vi "read position.vi"(8 "error in (no error)":errorcluster, 11 "CL57RS in":refnum<class "CL57RS.lvclass">) -> (0 "error out":errorcluster, 2 "Angle":dbl, 3 "CL57RS out":refnum<class "CL57RS.lvclass">)   [LabVIEW 2025, in "Motor.lvlib" / "CL57RS.lvclass"]
uses:
  CL57RS.lvclass
  CL57RS.lvclass/CL57RS.ctl
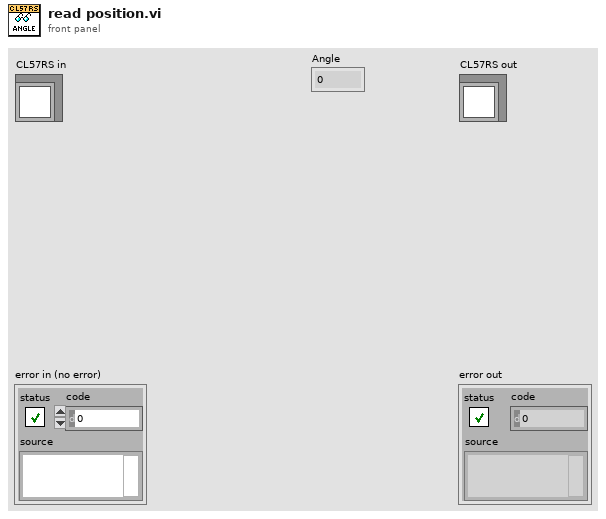
[diagram p1: front panel]
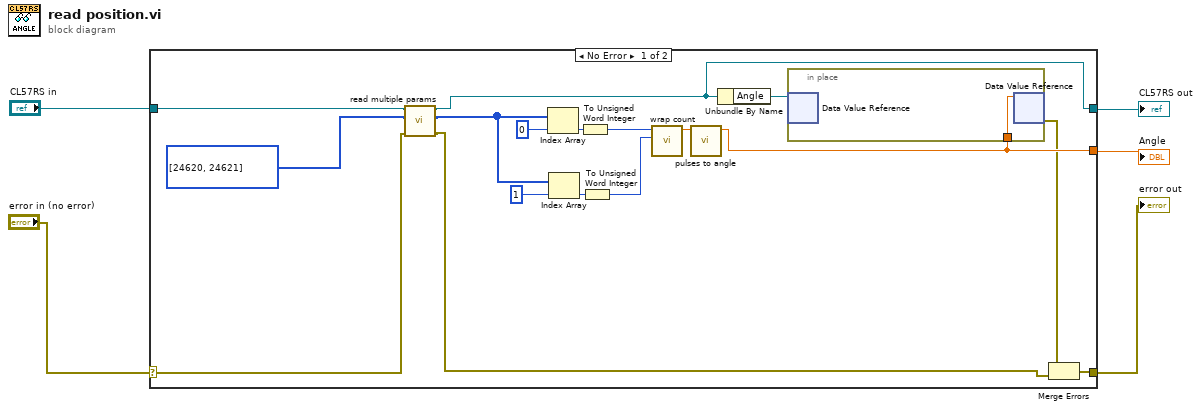
[diagram p0: block diagram]
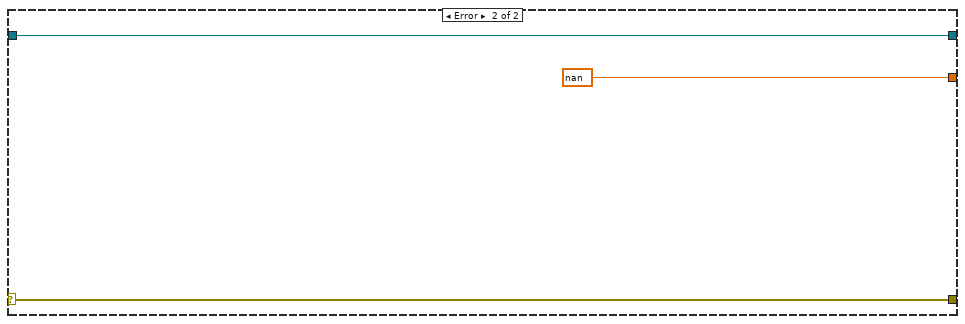
[diagram p2: hidden frame]
diagram:
  n1 = case shown="No Error" "error in (no error)" {
    selector: "error in (no error)" -> [w18 w26]
    tunnel: [w8 w26] -> w2
    tunnel: [w11 w25] -> w4
    tunnel: "CL57RS in" -> [w15 w25]
    tunnel: [w9 nan ("Angle")] -> w1
    frame No Error {
      n2 = call "read multiple params.vi"("error in (no error)"=w18, "Parameters"=u32[] [24620, 24621], "CL57RS in"=w15) -> ("error out"=w6:errorcluster, "Hex Result"=w16:u32[], "CL57RS out"=w11:refnum<class "CL57RS.lvclass">)  [unwired: 6 in]
      n3 = Index Array(array=w16, index=0) -> (element=w19:u32)
      n4 = Index Array(array=w16, index=1) -> (element=w20:u32)
      n5 = To Unsigned Word Integer(number=w19) -> (unsigned 16bit integer=w14:u16)
      n6 = To Unsigned Word Integer(number=w20) -> (unsigned 16bit integer=w13:u16)
      n7 = call "wrap count.vi"("lo"=w13, "hi"=w14) -> ("Numeric"=w12:dbl)  [unwired: 9 in]
      n8 = call "pulses to angle.vi"("Pulses"=w12) -> ("Angle"=w9:dbl)  [unwired: 10 in]
      n9 = Unbundle By Name(w11) -> ("Angle"=w10:refnum<data-value>)
      n10 = in-place {
        in-place-border: w9 -> [w23]
        n11 = in-place-dvr #1(w10) -> ()  [unwired: 2 out]
        n12 = in-place-dvr #1(w23) -> (w7:errorcluster)  [unwired: 1 out]
      }
      n13 = Merge Errors(w7, w6) -> (w8:errorcluster)
    }
    frame Error {
    }
  }
  "error out" <- w2
  "CL57RS out" <- w4
  "Angle" <- w1
